vi "Current Status Change.vi"(7 "Agilent Read Channels Array":T2[](array[typedef]), 8 "Test State":T1, 9 "Station Index":i32, 10 "Current Agilent Data":dbl[](array[numeric]), 11 "Dryer Status Serial Data In":T3) -> (3 "Dryer Status Serial Data In 2":T3)   [LabVIEW 2012]
uses:
  Dryer Com Port Info.ctl
  Dryer Status Ctrl.ctl
  Agilent Channel Definition.ctl
  Dryer Test State.ctl
  Globals Wilt.vi
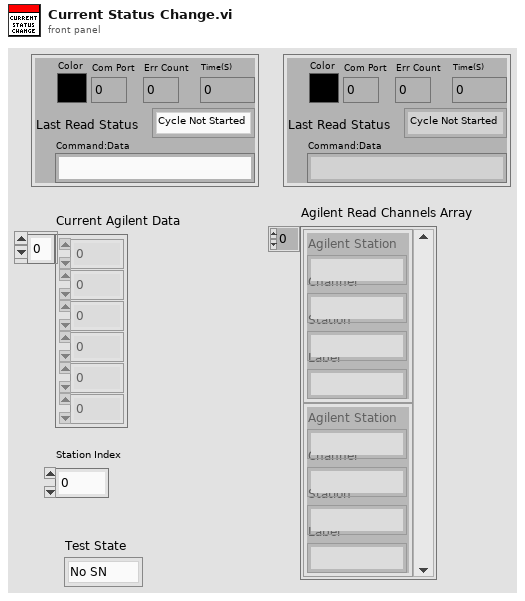
[diagram p1: front panel]
types:
  T1 = typedef "Dryer Test State.ctl" = enum16{"No SN", "Wait Com", "Wait to Start", "Watering", "Drying", "Cooldown", "Paused", "Temp Fault", "Com Fault", "Pause Manual Station"}
  T2 = typedef "Agilent Channel Definition.ctl" = cluster{"Channel":string, "Station":string, "Label":string, "Agilent Station":string}
  T3 = typedef "Dryer Com Port Info.ctl" = cluster{"Color":u32, "Last Read Status":T4, "Command:Data":string, "Com Port":u8, "Time(S)":dbl, "Err Count":u32}
  T4 = typedef "Dryer Status Ctrl.ctl" = enum16{"Cycle Not Started", "Cycle Running", "Paused", "Cycle Completed", "Eval Mode Entered", "Err", "Pause (No GEA2)"}
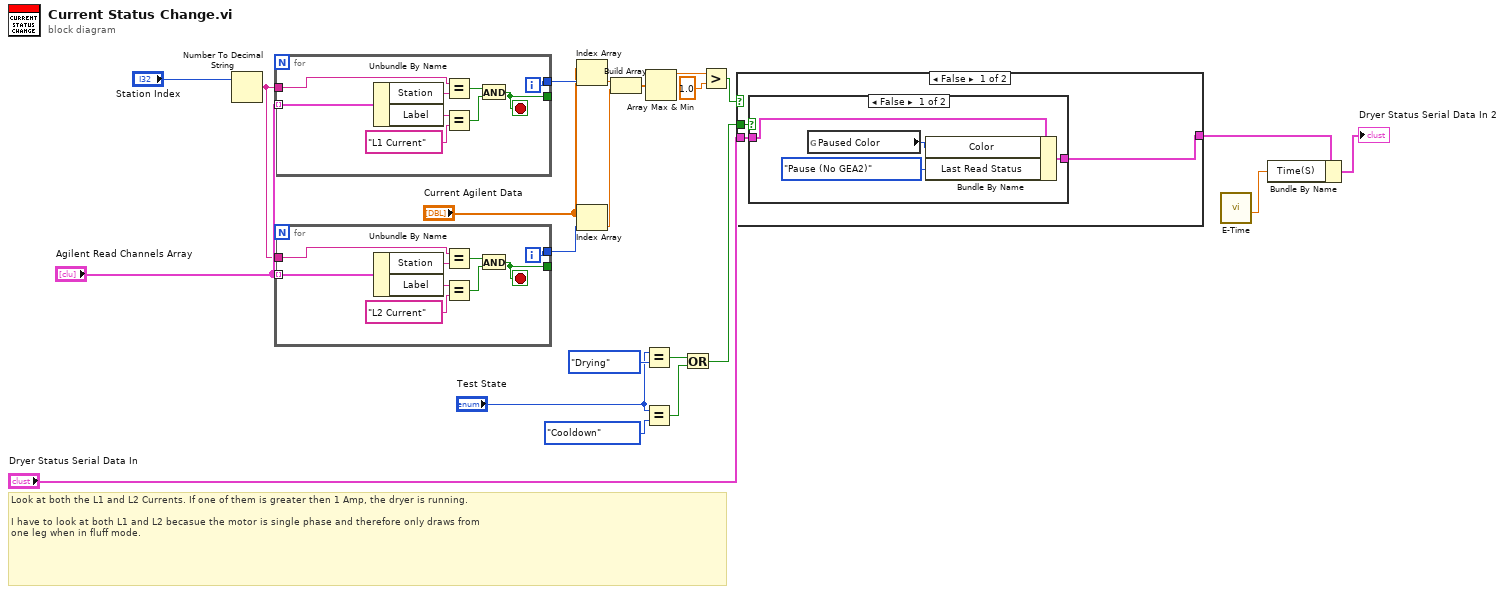
[diagram p0: block diagram]
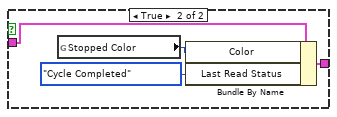
[diagram p2: hidden frame]
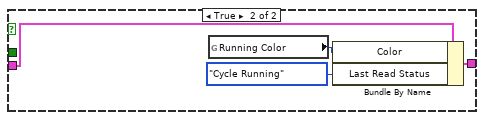
[diagram p3: hidden frame]
diagram:
  # "Look at both the L1 and L2 Currents. If one of them is greater then 1 Amp, the dryer is running.\n\nI have to look at both L1 and L2 becasue the motor is single phase and therefore only draws from\none leg when in fluff mode."
  n1 = Number To Decimal String(number="Station Index") -> (decimal integer string=w20:string)  [unwired: 1 in]
  n2 = for {
    tunnel: "Agilent Read Channels Array" -> [w31] mode=indexing
    tunnel: w20 -> [w26]
    tunnel: [w24] -> _
    tunnel: [w23] -> w19
    i -> [w23]
    stop <- w24 stop-if-true
    n3 = Unbundle By Name(w31) -> ("Station"=w27:string, "Label"=w30:string)
    n4 = Equal?(x=w26, y=w27) -> (x = y?=w25:bool)
    n5 = Equal?(x=w30, y="L1 Current") -> (x = y?=w28:bool)
    n6 = And(x=w25, y=w28) -> (x .and. y?=w24:bool)
  }
  n7 = for {
    tunnel: "Agilent Read Channels Array" -> [w40] mode=indexing
    tunnel: w20 -> [w35]
    tunnel: [w33] -> _
    tunnel: [w32] -> w18
    i -> [w32]
    stop <- w33 stop-if-true
    n8 = Unbundle By Name(w40) -> ("Station"=w36:string, "Label"=w39:string)
    n9 = Equal?(x=w35, y=w36) -> (x = y?=w34:bool)
    n10 = Equal?(x=w39, y="L2 Current") -> (x = y?=w37:bool)
    n11 = And(x=w34, y=w37) -> (x .and. y?=w33:bool)
  }
  n12 = Index Array(array="Current Agilent Data", index=w19) -> (element=w16:dbl)
  n13 = Index Array(array="Current Agilent Data", index=w18) -> (element=w15:dbl)
  n14 = Build Array(w16, w15) -> (w14:dbl[])
  n15 = Equal?(x="Test State", y=Dryer_Test_State."Drying" ("Test State")) -> (x = y?=w6:bool)
  n16 = Equal?(x="Test State", y=Dryer_Test_State."Cooldown" ("Test State")) -> (x = y?=w5:bool)
  n17 = Array Max & Min(array=w14) -> (max value=w12:dbl)  [unwired: 3 out]
  n18 = Or(x=w6, y=w5) -> (x .or. y?=w4:bool)
  n19 = Greater?(x=w12, y=1.0) -> (0:w11:bool)
  n20 = case shown="False" w11 {
    tunnel: "Dryer Status Serial Data In" -> [w43 w54]
    tunnel: [w42 w53] -> w3
    tunnel: w4 -> [w41 _]
    frame False {
      n21 = case shown="False" w41 {
        tunnel: w43 -> [w45 w51]
        tunnel: [w44 w50] -> w42
        frame False {
          n22 = global read "Globals Wilt.vi" "Paused Color"() -> (w47:u32)
          n23 = Bundle By Name(cluster=w45, "Color"=w47, "Last Read Status"=Dryer_Status_Ctrl."Pause (No GEA2)") -> (w44:T3)
        }
        frame True {
          n24 = global read "Globals Wilt.vi" "Stopped Color"() -> (w49:u32)
          n25 = Bundle By Name(cluster=w51, "Color"=w49, "Last Read Status"=Dryer_Status_Ctrl."Cycle Completed") -> (w50:T3)
        }
      }
    }
    frame True {
      n26 = global read "Globals Wilt.vi" "Running Color"() -> (w55:u32)
      n27 = Bundle By Name(cluster=w54, "Color"=w55, "Last Read Status"=Dryer_Status_Ctrl."Cycle Running") -> (w53:T3)
    }
  }
  n28 = call "E-Time.vi"() -> ("Elapsed Time (sec)"=w1:dbl)  [unwired: 9 in, 2 out]
  n29 = Bundle By Name(cluster=w3, "Time(S)"=w1) -> (→"Dryer Status Serial Data In 2":T3)
